vi "Commit History Parsing.vi"(8 "Error in":errorcluster caption="Error in (no error)", 11 "Commit History csv":path) -> (0 "Error out":errorcluster, 3 "File Change Map":T1 {"File Change Info"."Timestamp" format="%<%.0X %x>T"})   [LabVIEW 2023]
uses:
  TypeDefs/File Change Map.ctl
  <vilib>/Utility/miscctls.llb/LVMapReplaceAction.ctl
  <vilib>/Utility/file.llb/Read Delimited Spreadsheet (string).vi
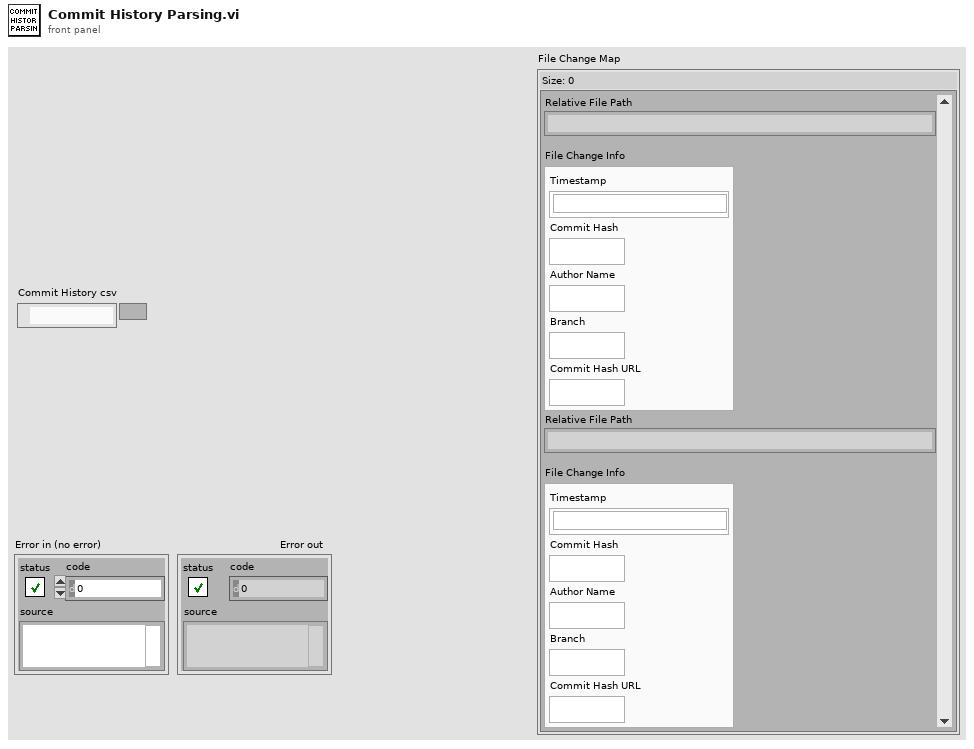
[diagram p1: front panel]
types:
  T1 = typedef "File Change Map.ctl" = map{string, cluster{"Timestamp":timestamp, "Commit Hash":string, "Author Name":string, "Branch":string, "Commit Hash URL":string}}
  T2 = typedef "LVMapReplaceAction.ctl" = enum32{"Modify Entry only if found", "Add or Modify Entry", "Delete Entry"}
  T3 = cluster{"Timestamp":timestamp, "Commit Hash":string, "Author Name":string, "Branch":string, "Commit Hash URL":string}
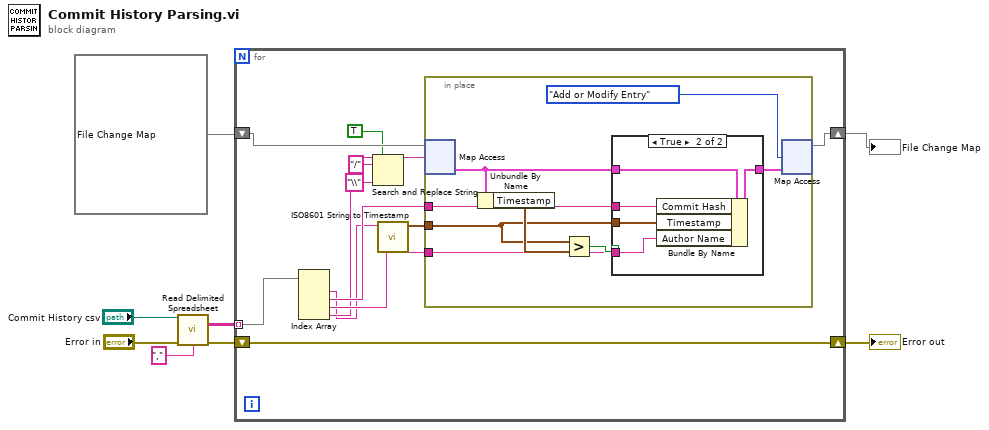
[diagram p0: block diagram]
diagram:
  n1 = call-poly <vilib>:"Read Delimited Spreadsheet.vi"("file path (dialog if empty)"="Commit History csv", "error in (no error)"="Error in", "delimiter (\\t)"="," ("delimiter (\\t)")) -> ("all rows"=w4:string[][], "error out"=w5:errorcluster)  [unwired: 7 in, 4 out]
  n2 = for {
    shift-right: [w9] -> w3
    shift-left: w5 -> [w9]
    tunnel: w4 -> [w21] mode=indexing
    shift-right: [w19] -> w2
    shift-left: T1 {} ("File Change Map") -> [w20]
    n3 = Index Array(array=w21) -> (element #1=w11:string, element #2=w18:string, element #3=w17:string, element #4=w15:string)  [unwired: 4 in]
    n4 = Search and Replace String(replace all?=TRUE ("replace all? (F)"), input string=w15, search string="/", replace string="\\" ("replace string (\"\")")) -> (result string=w16:string)  [unwired: 4 in, 3 out]
    n5 = call <vilib>:"ISO8601 String to Timestamp.vi"("ISO8601 String"=w11) -> ("Timestamp"=w10:timestamp)  [unwired: 8 in, 2 out]
    n6 = in-place {
      in-place-border: w10 -> [w24]
      in-place-border: w18 -> [w23]
      in-place-border: w17 -> [w22]
      n7 = in-place-map #1(w20, w16) -> (w28:T3)  [unwired: 1 in, 1 out]
      n8 = Unbundle By Name(w28) -> ("Timestamp"=w26:timestamp)
      n9 = Greater?(x=w24, y=w26) -> (0:w25:bool)
      n10 = case shown="True" w25 {
        tunnel: w28 -> [w30 w35]
        tunnel: [w30 w34] -> w27
        tunnel: w24 -> [_ w33]
        tunnel: w23 -> [_ w32]
        tunnel: w22 -> [_ w31]
        frame False {
        }
        frame True {
          n11 = Bundle By Name(cluster=w35, "Commit Hash"=w32, "Timestamp"=w33, "Author Name"=w31) -> (w34:T3)
        }
      }
      n12 = in-place-map #1(w27, LVMapReplaceAction."Add or Modify Entry" ("action")) -> (w19:T1)  [unwired: 2 out]
    }
  }
  "Error out" <- w3
  "File Change Map" <- w2
